vi "SFID_Close serial port.vi"(8 "Error in":errorcluster, 11 "VISA resource name":refnum<visa-resource-name>) -> (0 "Error out":errorcluster)   [LabVIEW 2022 SP3]
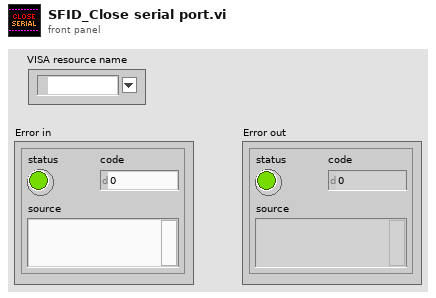
[diagram p1: front panel]
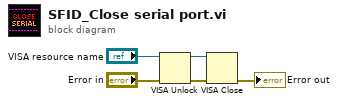
[diagram p0: block diagram]
diagram:
  n1 = VISA Unlock(8:"Error in", 11:"VISA resource name") -> (0:w1:errorcluster, 3:w3:refnum<visa-resource-name>)
  n2 = VISA Close(VISA resource name=w3, error in (no error)=w1) -> (error out=→"Error out":errorcluster)
